vi "SingleAcquisitionSaveTiffImage.vi"() -> ()   [LabVIEW 2018]
uses:
  C:/Users/Public/Documents/Photometrics/PMQI-LabViewSamples/Examples/Dependencies/PVCamNET.dll
  Public/Documents/Photometrics/PMQI-LabViewSamples/Examples/Dependencies/PVCamNET.dll
panel:
  out "Boolean 2":bool
  out "Boolean":bool
  in  "?":bool
  in  "?":bool
  in  "Exposure time":dbl=30.0
  in  "?":bool
  # "SingleAcqusitionSaveTiffImage.vi\n\nDescription:\nThis sample code lets the user use sequence mode and save a TIFF image with \nthe user's preferred exposure time. \n\nSteps to run:\n1. Click \"Run\"\n2. Enter Exposure time\n3. Click \"START\"\n4. Click \"SAVE\"\n5. Click \"CLOSE\""
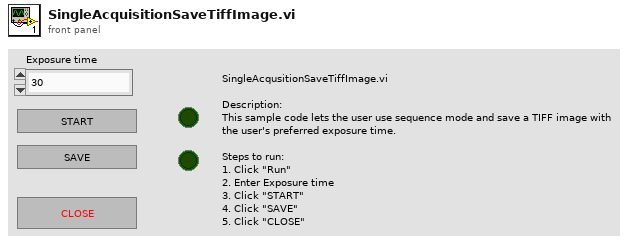
[diagram p1: front panel]
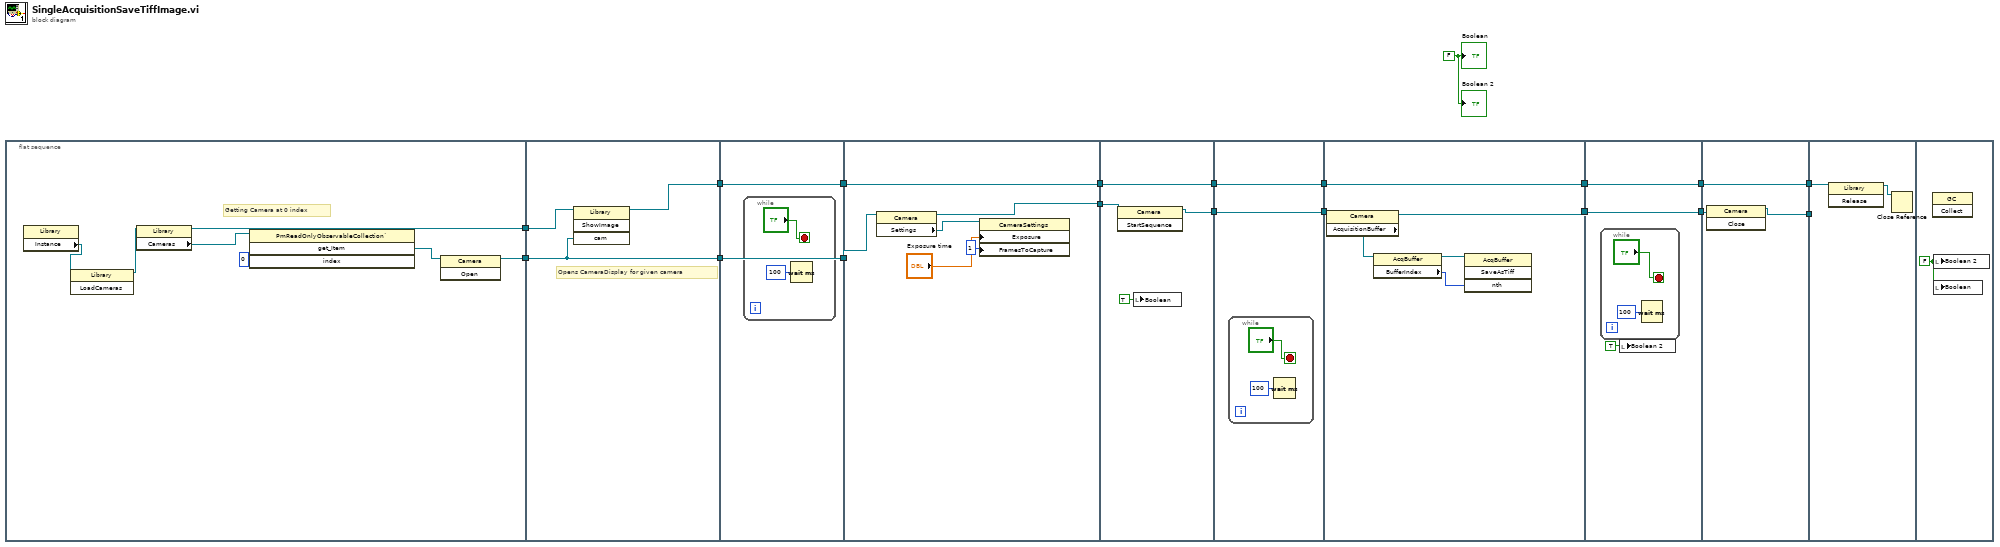
[diagram p0: block diagram]
diagram:
  w3 = FALSE ("Boolean")
  n1 = flat-sequence {
    tunnel: [w22] -> w19
    tunnel: [w23] -> w18
    tunnel: w19 -> [w29]
    tunnel: w18 -> [w28]
    tunnel: [w28] -> w17
    tunnel: [w27] -> w16
    tunnel: w17 -> [w31]
    tunnel: [w31] -> w14
    tunnel: w16 -> [w30]
    tunnel: [w30] -> w15
    tunnel: [w39] -> w13
    tunnel: [w38] -> w12
    tunnel: w15 -> [w38]
    tunnel: w14 -> [w37]
    tunnel: w13 -> [w42]
    tunnel: [w41] -> w7
    tunnel: [w43] -> w5
    tunnel: w12 -> [w43]
    tunnel: w7 -> [w45]
    tunnel: [w45] -> w6
    tunnel: w5 -> [w44]
    tunnel: [w44] -> w4
    tunnel: w6 -> [w52]
    tunnel: [w50] -> w2
    tunnel: w4 -> [w53]
    tunnel: [w53] -> w1
    tunnel: w2 -> [w56]
    tunnel: [w56] -> w9
    tunnel: w1 -> [w55]
    tunnel: [w55] -> w8
    tunnel: w9 -> [w61]
    tunnel: w8 -> [w59]
    tunnel: [w60] -> w11
    tunnel: [w59] -> w10
    tunnel: w11 -> [_]
    tunnel: w10 -> [w63]
    frame #0 {
      # "Getting Camera at 0 index"
      n2 = property class="Library"() -> ("Instance"=w21:refnum<k24>)  [unwired: 2 in, 2 out]
      n3 = invoke class="Library" method="LoadCameras"(reference=w21) -> (reference out=w20:refnum<k24>)  [unwired: 2 in, 2 out]
      n4 = property class="Library"(reference=w20) -> (reference out=w22:refnum<k24>, "Cameras"=w26:refnum<k24>)  [unwired: 1 in, 1 out]
      n5 = invoke class="PmReadOnlyObservableCollection`" method="get_Item"(reference=w26, "index"=0) -> ("get_Item"=w24:refnum<k24>)  [unwired: 2 in, 3 out]
      n6 = invoke class="Camera" method="Open"(reference=w24) -> (reference out=w23:refnum<k24>)  [unwired: 2 in, 2 out]
    }
    frame #1 {
      # "Opens CameraDisplay for given camera"
      n7 = invoke class="Library" method="ShowImage"(reference=w29, "cam"=w28) -> (reference out=w27:refnum<k24>)  [unwired: 2 in, 3 out]
    }
    frame #2 {
      n8 = while {
        stop <- "?" stop-if-true
        n9 = Wait (ms)(milliseconds to wait=u32 100) -> ()  [unwired: 1 out]
      }
    }
    frame #3 {
      n10 = property class="Camera"(reference=w37) -> (reference out=w39:refnum<k24>, "Settings"=w35:refnum<k24>)  [unwired: 1 in, 1 out]
      n11 = property class="CameraSettings"(reference=w35, "Exposure"="Exposure time", "FramesToCapture"=u16 1) -> ()  [unwired: 1 in, 2 out]
    }
    frame #4 {
      n12 = invoke class="Camera" method="StartSequence"(reference=w42) -> (reference out=w41:refnum<k24>)  [unwired: 2 in, 2 out]
      n13 = local write "Boolean"(TRUE ("Boolean")) -> ()
    }
    frame #5 {
      n14 = while {
        stop <- "?" stop-if-true
        n15 = Wait (ms)(milliseconds to wait=u32 100) -> ()  [unwired: 1 out]
      }
    }
    frame #6 {
      n16 = property class="Camera"(reference=w52) -> (reference out=w50:refnum<k24>, "AcquisitionBuffer"=w51:refnum<k24>)  [unwired: 1 in, 1 out]
      n17 = property class="AcqBuffer"(reference=w51) -> (reference out=w49:refnum<k24>, "BufferIndex"=w48:i32)  [unwired: 1 in, 1 out]
      n18 = invoke class="AcqBuffer" method="SaveAsTiff"(reference=w49, "nth"=w48) -> ()  [unwired: 2 in, 4 out]
    }
    frame #7 {
      n19 = while {
        stop <- "?" stop-if-true
        n20 = Wait (ms)(milliseconds to wait=u32 100) -> ()  [unwired: 1 out]
      }
      n21 = local write "Boolean 2"(TRUE ("Boolean 2")) -> ()
    }
    frame #8 {
      n22 = invoke class="Camera" method="Close"(reference=w61) -> (reference out=w60:refnum<k24>)  [unwired: 2 in, 2 out]
    }
    frame #9 {
      n23 = invoke class="Library" method="Release"(reference=w63) -> (reference out=w62:refnum<k24>)  [unwired: 2 in, 2 out]
      n24 = Close Reference(reference=w62) -> ()  [unwired: 1 in, 1 out]
    }
    frame #10 {
      w64 = FALSE ("Boolean 2")
      n25 = invoke class="GC" method="Collect"() -> ()  [unwired: 3 in, 3 out]
      n26 = local write "Boolean 2"(w64) -> ()
      n27 = local write "Boolean"(w64) -> ()
    }
  }
  "Boolean" <- w3
  "Boolean 2" <- w3
